vi "Read Analogue.vi"(8 "error in (no error)":errorcluster, 11 "Sim PS in":refnum<class "Sim PS.lvclass">) -> (0 "error out":errorcluster, 2 "Measurement":dbl, 3 "Sim PS out":refnum<class "Sim PS.lvclass">)   [LabVIEW 2019, in "Concrete.lvlib" / "Sim PS.lvclass"]
uses:
  Sim PS.lvclass
  <vilib>/numeric/Random Number (Range) DBL.vi
  Harware Abstraction/Analog out/Analog out.lvclass
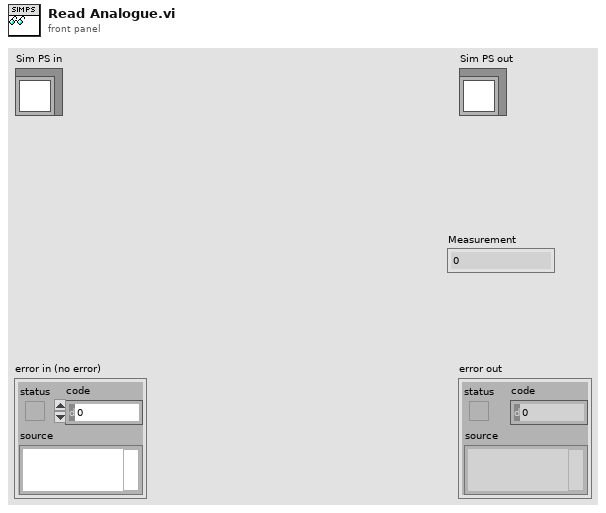
[diagram p1: front panel]
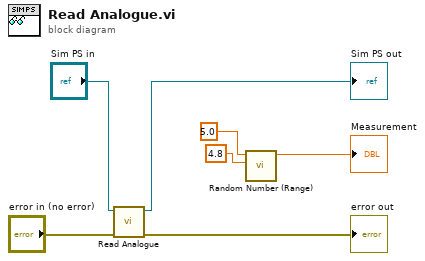
[diagram p0: block diagram]
diagram:
  n1 = call-parent "Read Analogue.vi"("error in (no error)"="error in (no error)", "Analog out in"="Sim PS in") -> ("error out"=→"error out":errorcluster, "Analog out out"=→"Sim PS out":refnum<class "Sim PS.lvclass">)  [unwired: 7 in, 1 out]
  n2 = call-poly <vilib>:"Random Number (Range).vi"("lower bound (0)"=4.8, "upper bound (100)"=5.0) -> ("number"=→"Measurement":dbl)  [unwired: 9 in]
